vi "Set Float Parameter.vi"(8 "error in (no error)":errorcluster, 9 "Value":sgl, 10 "Parameter Name":string, 11 "VoiceMeeterRemote in":refnum<class "VoiceMeeterRemote.lvclass">) -> (0 "error out":errorcluster, 3 "VoiceMeeterRemote out":refnum<class "VoiceMeeterRemote.lvclass">)   [LabVIEW 2022 SP3, in "VoiceMeeterRemote.lvlib" / "VoiceMeeterRemote.lvclass"]
uses:
  VoiceMeeterRemote.lvclass
  VoiceMeeterRemote.lvclass/VoiceMeeterRemote.ctl
  VoiceMeeterRemote.lvlib
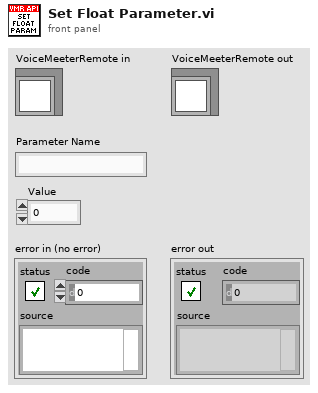
[diagram p1: front panel]
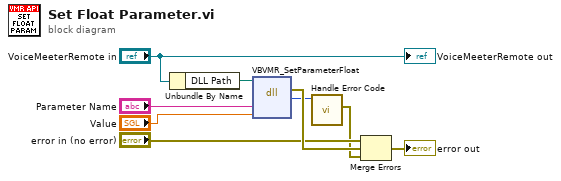
[diagram p0: block diagram]
diagram:
  n1 = Unbundle By Name("VoiceMeeterRemote in") -> ("DLL Path"=w7:path)
  n2 = dll-call lib="C:/Program Files/National Instruments/LabVIEW 2022/user.lib/VoicemeeterRemote64/VoicemeeterRemote64.*" fn="VBVMR_SetParameterFloat"(path in=w7, "szParamName"="Parameter Name", "Value"="Value") -> (error out=w9:errorcluster, "return type"=w4:i32)  [unwired: 4 in, 1 out]
  n3 = call "Handle Error Code.vi"("Code"=w4) -> ("error out"=w2:errorcluster)  [unwired: 10 in]
  n4 = Merge Errors("error in (no error)", w9, w2) -> (→"error out":errorcluster)
  "VoiceMeeterRemote out" <- "VoiceMeeterRemote in"
